vi "PRIME Detector Pipeline Check Status for New Files.vi"(5 "Observation":T2={"Priority"=0, "ID"="", "Observer"="", "Obj Name"="", "Obj Type"="", "RA and DEC String"={"RA"="HH:MM:SS.nnn", "DEC"="DEG:arcmin:arcsec.nn"}, "Filters"=[], "Integration Time"=0.0, "Observation Status"=enum."Error", "Offsets"={"RA"=0.0, "DEC"=0.0, "ROT"=0.0}, "Images"=0, "Dither Options"={"Dither"=enum."None", "Dither Radius"=0.0, "Dither Points"=0, "Dither Phase"=0.0, "B Offset"={"RA"=0.0, "DEC"=0.0}}, "Comment 1"="", "Comment 2"=""}, 7 "Detector Config":T8={"Detector"=0, "Offsets"=[[0, 0, 0, 0, 0, 0, 0, 0, 0, 0, 0, 0, 0, 0, 0, 0, 0, 0, 0, 0, 0, 0, 0, 0, 0, 0, 0, 0, 0, 0, 0, 0]], "Detector Computer"={"Machine"="192.168.121.11", "Password"="rSL!nux23456", "FITS File Path"="", "Port"=44444, "Header Path"="", "Name"=""}, "FITS hdr template0"=path "", "FITS hdr template1"=path "", "FITS Data File Path"=path "", "FITS Detector Settings"={"Exp Time Short"=0.0, "# of Frames"=0.0, "Exp Time Long"=0.0, "# of Groups"=0.0, "Object Name"="", "Object"="", "Obs Type"="", "Image Type"="", "Observer"="", "Observer Affiliation"=""}, "Sim Folder"=path "", "Integration Mode"=enum."Ramp", "Integration Time"=0.0, "Frame Int Time"=0.0} {"Offsets" format="%04x"; "Detector" items=["0", "1", "2"]}, 8 "error in (no error)":errorcluster, 10 "Status":T1, 11 "Map in":map{string, T12}(c390)) -> (0 "error out":errorcluster, 3 "Map out":map{string, T12}(c390))   [LabVIEW 2024]
uses:
  Detector Image typedef cluster.ctl
  RIMAS Detector Config.ctl
  RIMAS Detector Server Config.ctl
  RIMAS Observation Config.ctl
  Detector enum Detector Integration Mode.ctl
  typedefs/CC cluster Observation.ctl
  Observation Queue/CC enum Observation Status.ctl
  Telescope/CC cluster Telescope Offsets.ctl
  typedefs/CC cluster Observation Dither Options.ctl
  typedefs/CC enum Dither Selection.ctl
  typedefs/CC cluster RA and DEC.ctl
  PRIME Detector cluster Status.ctl
  Detector Class.lvclass
panel:
  # "sec"
  # "sec"
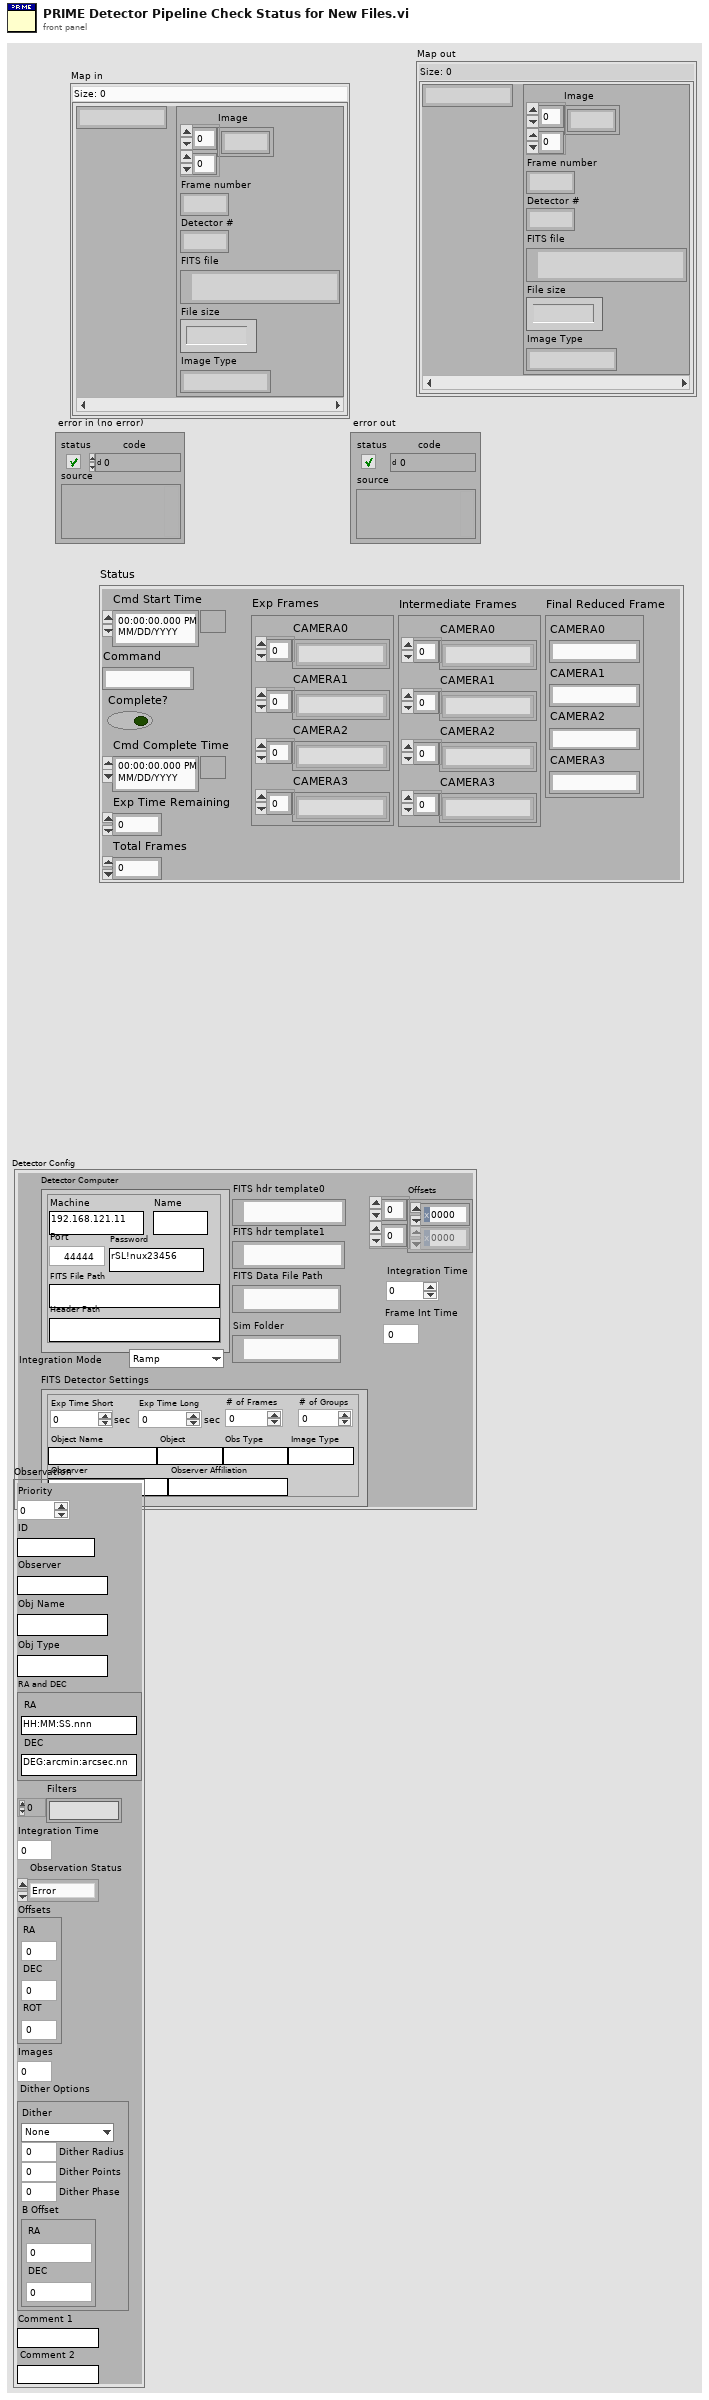
[diagram p1: front panel]
types:
  T1 = typedef "PRIME Detector cluster Status.ctl" = cluster{"Cmd Start Time":timestamp, "Command":string, "Complete?":bool, "Cmd Complete Time":timestamp, "Exp Time Remaining":dbl, "Total Frames":i32, "Exp Frames":cluster{"CAMERA0":string[], "CAMERA1":string[], "CAMERA2":string[], "CAMERA3":string[]}, "Intermediate Frames":cluster{"CAMERA0":string[], "CAMERA1":string[], "CAMERA2":string[], "CAMERA3":string[]}, "Final Reduced Frame":cluster{"CAMERA0":string, "CAMERA1":string, "CAMERA2":string, "CAMERA3":string}}
  T2 = typedef "CC cluster Observation.ctl" = cluster{"Priority":i32, "ID":string, "Observer":string, "Obj Name":string, "Obj Type":string, "RA and DEC String":cluster{"RA":string, "DEC":string}, "Filters":string[], "Integration Time":dbl, "Observation Status":T3, "Offsets":T4, "Images":i32, "Dither Options":T5, "Comment 1":string, "Comment 2":string}
  T3 = typedef "CC enum Observation Status.ctl" = enum16{"Ready", "Running", "Done", "Error"}
  T4 = typedef "CC cluster Telescope Offsets.ctl" = cluster{"RA":dbl, "DEC":dbl, "ROT":dbl}
  T5 = typedef "CC cluster Observation Dither Options.ctl" = cluster{"Dither":T6, "Dither Radius":dbl, "Dither Points":i32, "Dither Phase":dbl, "B Offset":T7}
  T6 = typedef "CC enum Dither Selection.ctl" = enum16{"None", "Circle", "Random", "ABBA"}
  T7 = typedef "CC cluster RA and DEC.ctl" = cluster{"RA":dbl, "DEC":dbl}
  T8 = typedef "RIMAS Detector Config.ctl" = cluster{"Detector":u16, "Offsets":u16[][], "Detector Computer":T9, "FITS hdr template0":path, "FITS hdr template1":path, "FITS Data File Path":path, "FITS Detector Settings":T10, "Sim Folder":path, "Integration Mode":T11, "Integration Time":dbl, "Frame Int Time":dbl}
  T9 = typedef "RIMAS Detector Server Config.ctl" = cluster{"Machine":string, "Password":string, "FITS File Path":string, "Port":u16, "Header Path":string, "Name":string}
  T10 = typedef "RIMAS Observation Config.ctl" = cluster{"Exp Time Short":dbl, "# of Frames":dbl, "Exp Time Long":dbl, "# of Groups":dbl, "Object Name":string, "Object":string, "Obs Type":string, "Image Type":string, "Observer":string, "Observer Affiliation":string}
  T11 = typedef "Detector enum Detector Integration Mode.ctl" = enum16{"Ramp", "CDS", "FOWLER2", "FOWLER4", "FOWLER8", "FOWLER16", "Raw"}
  T12 = typedef "Detector Class.lvclass/Detector Image typedef cluster.ctl" = cluster{"Image":sgl[][], "Frame number":i32, "Detector #":u16, "FITS file":path, "File size":i64, "Image Type":string}
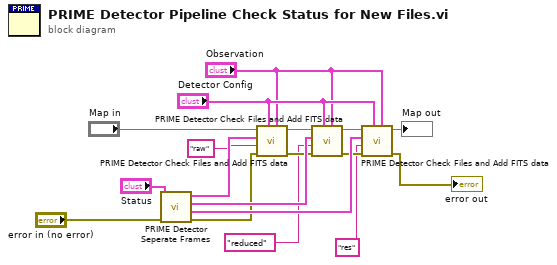
[diagram p0: block diagram]
diagram:
  n1 = call "PRIME Detector Seperate Frames.vi"("error in (no error)"="error in (no error)", "Status"="Status") -> ("error out"=w10:errorcluster, "Final Frames"=w14:cluster{string[]}[], "Inter Frames"=w15:cluster{"CAMERA3":string[]}[], "Exp Frames"=w18:cluster{"CAMERA3":string[]}[])  [unwired: 6 in]
  n2 = call "PRIME Detector Check Files and Add FITS data.vi"("Observation"="Observation", "Detector Config"="Detector Config", "error in (no error)"=w10, "Image Type"="raw", "Image Array"=w18, "Map in"="Map in") -> ("error out"=w9:errorcluster, "Map out"=w17:map{string, T12})  [unwired: 4 in]
  n3 = call "PRIME Detector Check Files and Add FITS data.vi"("Observation"="Observation", "Detector Config"="Detector Config", "error in (no error)"=w9, "Image Type"="reduced", "Image Array"=w15, "Map in"=w17) -> ("error out"=w8:errorcluster, "Map out"=w16:map{string, T12})  [unwired: 4 in]
  n4 = call "PRIME Detector Check Files and Add FITS data.vi"("Observation"="Observation", "Detector Config"="Detector Config", "error in (no error)"=w8, "Image Type"="res", "Image Array"=w14, "Map in"=w16) -> ("error out"=→"error out":errorcluster, "Map out"=→"Map out":map{string, T12})  [unwired: 4 in]
